vi "Find Class in Memory.vi"(11 "Class Name":string) -> (2 "Class Found?":bool, 3 "Full Class Name":string)   [LabVIEW 2014, in "PL Framework Configuration Tool.lvlib" / "SystemConfigRepo.lvclass"]
doc: "Search libraries currently loaded in memory for class name input. Class Name input must be in the form of *.lvclass.\n\nThis functionality is also used by class discovery singleton.lvlib:loadclass.vi"
uses:
  SystemConfigRepo.lvclass
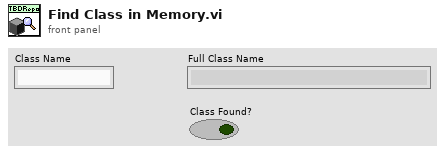
[diagram p1: front panel]
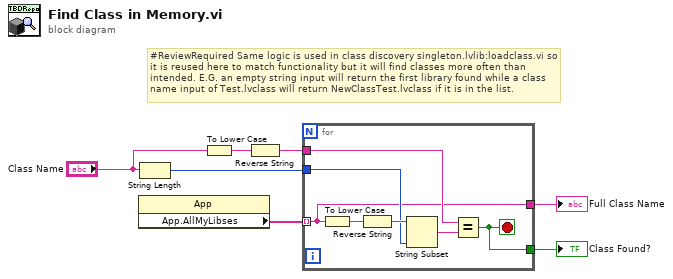
[diagram p0: block diagram]
diagram:
  # "#ReviewRequired Same logic is used in class discovery singleton.lvlib:loadclass.vi so it is reused here to match functionality but it will find classes more often than intended. E.G. an empty string input will return the first library found while a class name input of Test.lvclass will return NewClassTest.lvclass if it is in the list."
  n1 = property class="App"() -> ("App.AllMyLibses"=w2:string[])  [unwired: 2 in, 2 out]
  n2 = String Length(string="Class Name") -> (length=w3:i32)
  n3 = To Lower Case(string="Class Name") -> (all lower case string=w4:string)
  n4 = Reverse String(1:w4) -> (0:w5:string)
  n5 = for {
    tunnel: w2 -> [w8] mode=indexing
    tunnel: w5 -> [w14]
    tunnel: w3 -> [w12]
    tunnel: [w8] -> w6
    tunnel: [w10] -> w7
    stop <- w10 stop-if-true
    n6 = To Lower Case(string=w8) -> (all lower case string=w9:string)
    n7 = Reverse String(1:w9) -> (0:w13:string)
    n8 = String Subset(string=w13, length (rest)=w12) -> (substring=w11:string)  [unwired: 1 in]
    n9 = Equal?(x=w14, y=w11) -> (x = y?=w10:bool)
  }
  "Class Found?" <- w7
  "Full Class Name" <- w6
